vi "set_internal_files.vi"(8 "error in (no error)":errorcluster, 10 "number of channels":i32, 11 "pulse_gen_and_detect_p2p in":refnum<class "pulse_gen_and_detect_p2p.lvclass">) -> (0 "error out":errorcluster, 3 "pulse_gen_and_detect_p2p out":refnum<class "pulse_gen_and_detect_p2p.lvclass">)   [LabVIEW 2021, in "pulse_gen_and_detect_p2p.lvclass"]
uses:
  pulse_gen_and_detect_p2p.lvclass
  pulse_gen_and_detect_p2p.lvclass/pulse_gen_and_detect_p2p.ctl
  device_type/device_type.lvclass
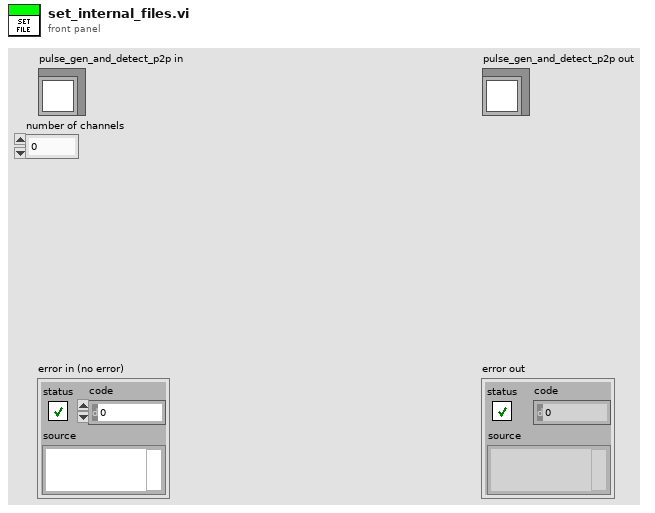
[diagram p1: front panel]
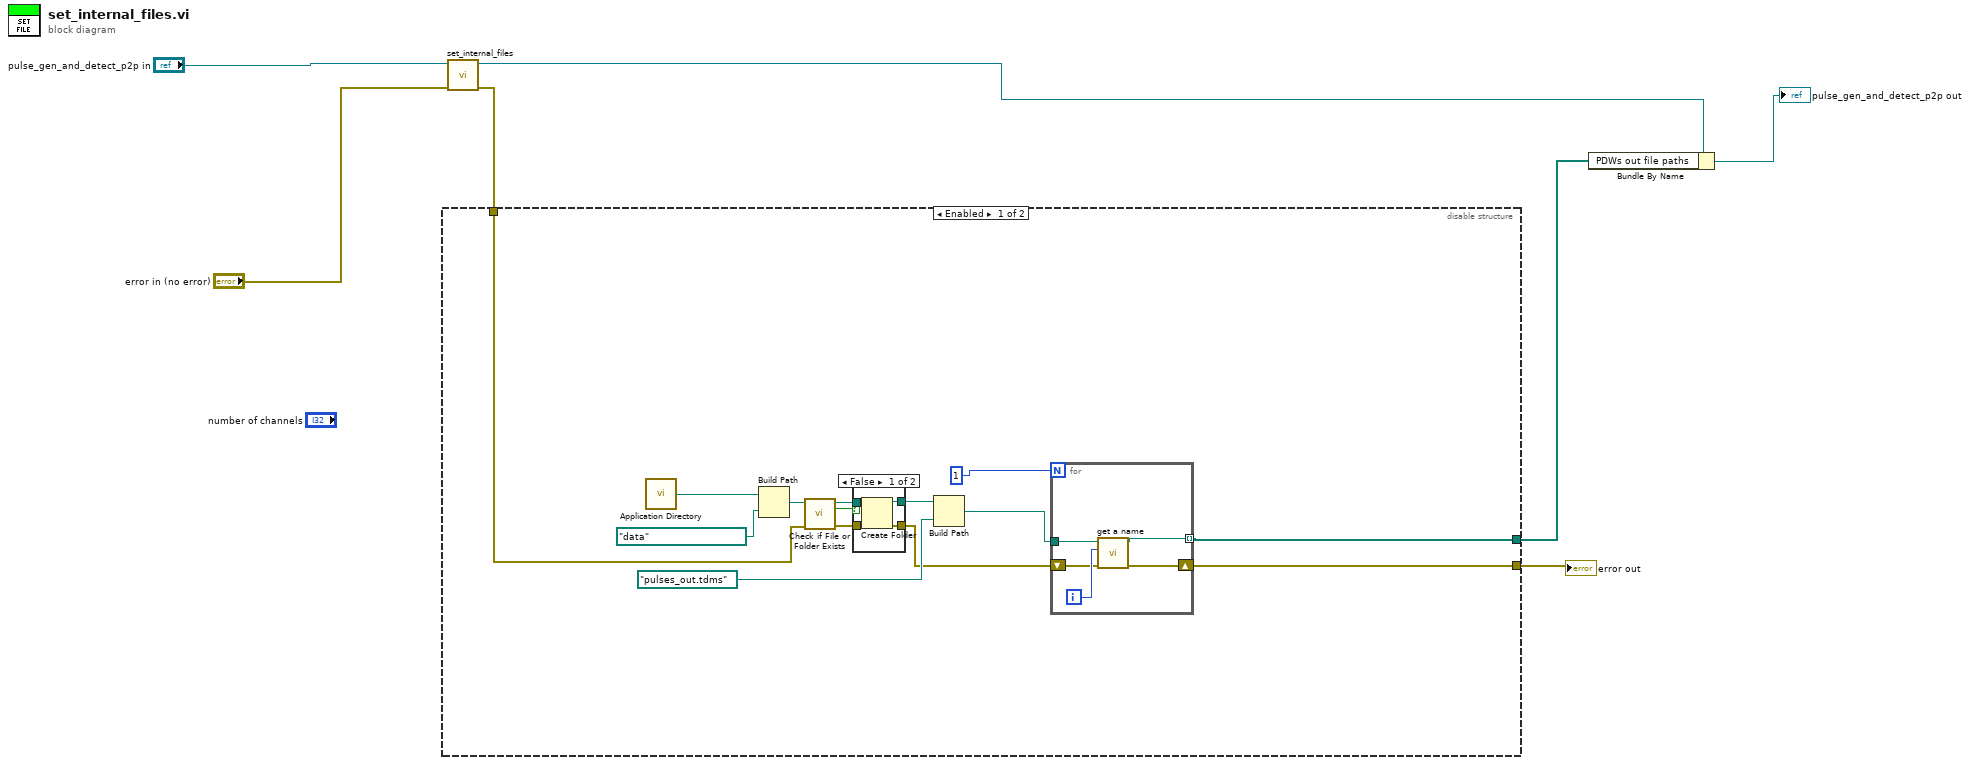
[diagram p0: block diagram]
diagram:
  n1 = call-parent "set_internal_files.vi"("error in (no error)"="error in (no error)", "device_type in"="pulse_gen_and_detect_p2p in") -> ("error out"=w5:errorcluster, "device_type out"=w3:refnum<class "pulse_gen_and_detect_p2p.lvclass">)  [unwired: 8 in]
  n2 = disable-structure shown="Enabled" {
    disable-tunnel: w5 -> [w10 w33]
    disable-tunnel: [w9 w33] -> w4
    disable-tunnel: [w8 _] -> w2
    frame Enabled {
      n3 = call <vilib>:"Application Directory.vi"() -> ("Application Directory"=w19:path)
      n4 = Build Path(base path=w19, name or relative path=path "data") -> (appended path=w16:path)
      n5 = call <vilib>:"Check if File or Folder Exists.vi"("error in (no error)"=w10, "path"=w16) -> ("error out"=w13:errorcluster, "file or folder exists?"=w11:bool, "dup path"=w15:path)  [unwired: 7 in]
      n6 = case shown="False" w11 {
        tunnel: w15 -> [w25 w27]
        tunnel: [w24 w27] -> w14
        tunnel: w13 -> [w23 w26]
        tunnel: [w22 w26] -> w12
        frame False {
          n7 = Create Folder(path (use dialog)=w25, error in=w23) -> (created path=w24:path, error out=w22:errorcluster)  [unwired: 1 in, 1 out]
        }
        frame True {
        }
      }
      n8 = Build Path(base path=w14, name or relative path=path "pulses_out.tdms") -> (appended path=w17:path)
      n9 = for {
        N: 1 -> [_]
        tunnel: w17 -> [w32]
        shift-right: [w29] -> w9
        shift-left: w12 -> [w30]
        tunnel: [w28] -> w8 mode=indexing
        i -> [w31]
        n10 = call "get a name.vi"("error constant"=w30, "Numeric"=w31, "Bitfile path"=w32) -> ("error constant 2"=w29:errorcluster, "Path"=w28:path)  [unwired: 7 in]
      }
    }
    frame Disabled {
    }
  }
  "error out" <- w4
  n11 = Bundle By Name(cluster=w3, "PDWs out file paths"=w2) -> (→"pulse_gen_and_detect_p2p out":refnum<class "pulse_gen_and_detect_p2p.lvclass">)
